vi "Set On State on Multiple Controls.vi"(10 "Enable?":bool caption="on?", 11 "Controls":refnum<vi>[](array[refnum]) caption="컨트롤") -> (3 "Controls 2":refnum<vi>[](array[refnum]) caption="컨트롤")   [LabVIEW 2018, in "Library-Ctrl.lvlib"]
doc: "입력 배열의 모든 컨트롤을 \"활성화 상태\" 값으로 설정합니다."
uses:
  Library-Ctrl.lvlib
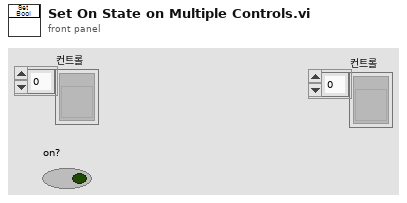
[diagram p1: front panel]
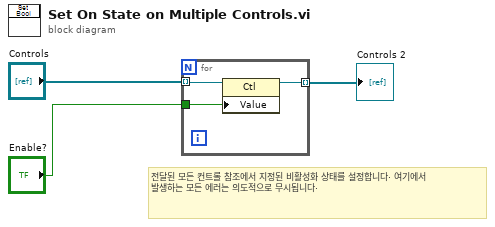
[diagram p0: block diagram]
diagram:
  # "전달된 모든 컨트롤 참조에서 지정된 비활성화 상태를 설정합니다. 여기에서 발생하는 모든 에러는 의도적으로 무시됩니다."
  n1 = for {
    tunnel: "Controls" -> [w6] mode=indexing
    tunnel: "Enable?" -> [w5]
    tunnel: [w4] -> w1 mode=indexing
    n2 = property class="Ctl"(reference=w6, "Value"=w5) -> (reference out=w4:refnum<vi>)  [unwired: 1 in, 1 out]
  }
  "Controls 2" <- w1
